vi "Solve1.vi"(8 "Error In":errorcluster, 11 "object in":refnum<class "2022_4.lvclass">) -> (0 "Error Out":errorcluster, 2 "Result":u64, 3 "object out":refnum<class "2022_4.lvclass">)   [LabVIEW 2020, in "2022_4.lvclass"]
uses:
  2022_4.lvclass
  2022_4.lvclass/2022_4.ctl
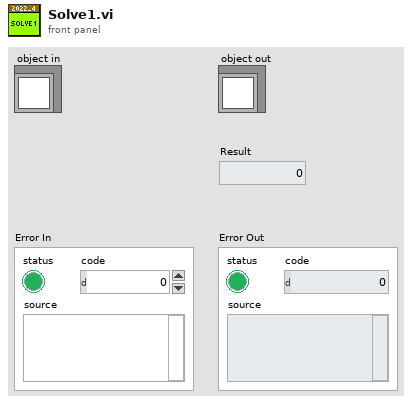
[diagram p1: front panel]
types:
  T1 = cluster{"Elf1":cluster{"Start":i32, "End":i32}, "Elf2":cluster{"Start":i32, "End":i32}}[]
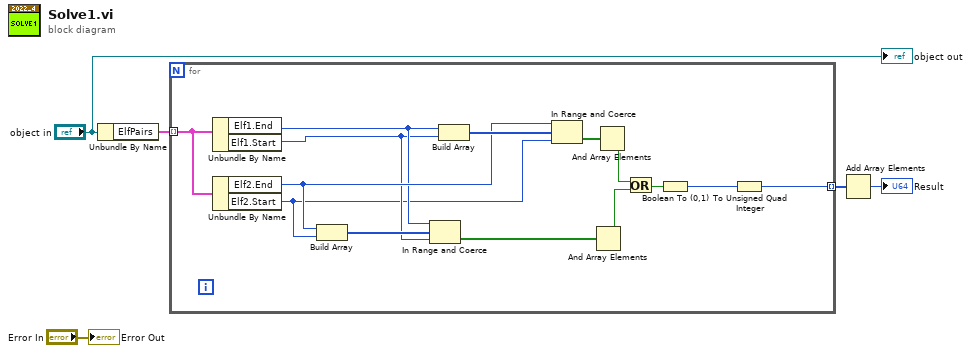
[diagram p0: block diagram]
diagram:
  n1 = Unbundle By Name("object in") -> ("ElfPairs"=w2:T1)
  n2 = for {
    tunnel: w2 -> [w19] mode=indexing
    tunnel: [w7] -> w1 mode=indexing
    n3 = Unbundle By Name(w19) -> ("Elf1.End"=w13:i32, "Elf1.Start"=w12:i32)
    n4 = Unbundle By Name(w19) -> ("Elf2.End"=w14:i32, "Elf2.Start"=w6:i32)
    n5 = Build Array(w14, w6) -> (w15:i32[])
    n6 = In Range and Coerce(upper limit=w13, x=w15, lower limit=w12) -> (In Range?=w16:bool[])  [unwired: 1 out]
    n7 = Build Array(w13, w12) -> (w18:i32[])
    n8 = In Range and Coerce(upper limit=w14, x=w18, lower limit=w6) -> (In Range?=w17:bool[])  [unwired: 1 out]
    n9 = And Array Elements(Boolean array=w16) -> (logical AND=w10:bool)
    n10 = And Array Elements(Boolean array=w17) -> (logical AND=w11:bool)
    n11 = Or(x=w11, y=w10) -> (x .or. y?=w9:bool)
    n12 = Boolean To (0,1)(Boolean=w9) -> (0, 1=w8:i16)
    n13 = To Unsigned Quad Integer(1:w8) -> (0:w7:u64)
  }
  n14 = Add Array Elements(numeric array=w1) -> (sum=→"Result":u64)
  "Error Out" <- "Error In"
  "object out" <- "object in"
